vi "Compressor.vi"(1 "Run":bool, 2 "Mode":enum8{"Start", "Run", "Finish"}(ring)) -> (0 "Compressor Running":bool)   [LabVIEW 2014]
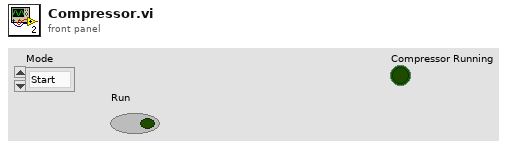
[diagram p1: front panel]
types:
  T1 = typedef "WPI_CompressorDevRef.ctl" = cluster{"DevStatus":errorcluster, "Pneumatics Control Module":u8}
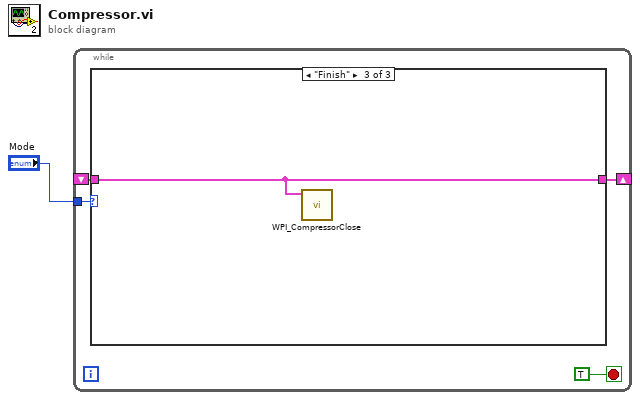
[diagram p0: block diagram]
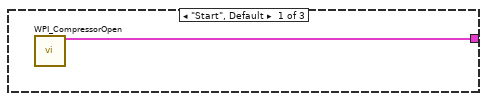
[diagram p2: hidden frame]
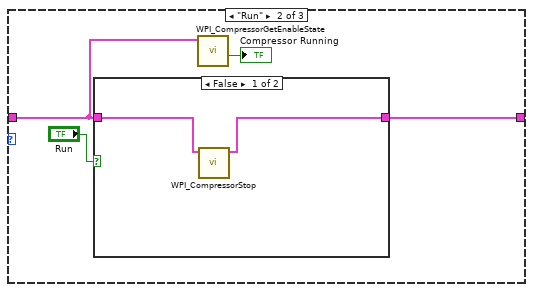
[diagram p3: hidden frame]
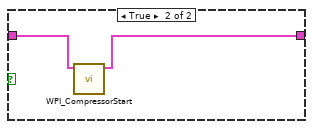
[diagram p4: hidden frame]
diagram:
  n1 = while {
    tunnel: "Mode" -> [w4]
    shift-right: [w3] -> _
    shift-left: _ -> [w2]
    stop <- TRUE stop-if-true
    n2 = case shown="\"Finish\"" w4 {
      tunnel: [w6 w9 w15] -> w3
      tunnel: w2 -> [_ w8 w15]
      frame "Start", Default {
        n3 = call <vilib>:"WPI_CompressorOpen.vi"() -> ("CompressorDevRef"=w6:T1)  [unwired: 14 in, 1 out]
      }
      frame "Run" {
        n4 = case shown="False" "Run" {
          tunnel: w8 -> [w12 w14]
          tunnel: [w11 w13] -> w9
          frame False {
            n5 = call <vilib>:"WPI_CompressorStop.vi"("CompressorDevRef"=w12) -> ("CompressorDevRef"=w11:T1)  [unwired: 9 in, 1 out]
          }
          frame True {
            n6 = call <vilib>:"WPI_CompressorStart.vi"("CompressorDevRef"=w14) -> ("CompressorDevRef"=w13:T1)  [unwired: 9 in, 1 out]
          }
        }
        n7 = call <vilib>:"WPI_CompressorGetEnableState.vi"("CompressorDevRef"=w8) -> ("Compressor Running"=→"Compressor Running":bool)  [unwired: 7 in, 3 out]
      }
      frame "Finish" {
        n8 = call <vilib>:"WPI_CompressorClose.vi"("CompressorDevRef"=w15) -> ()  [unwired: 10 in, 1 out]
      }
    }
  }
